vi "Solution Acquire Analyze Present.vi"() -> ()   [LabVIEW 2019]
panel:
  out "Difference":dbl
  out "Waveform Graph":dynamicdata(graph)
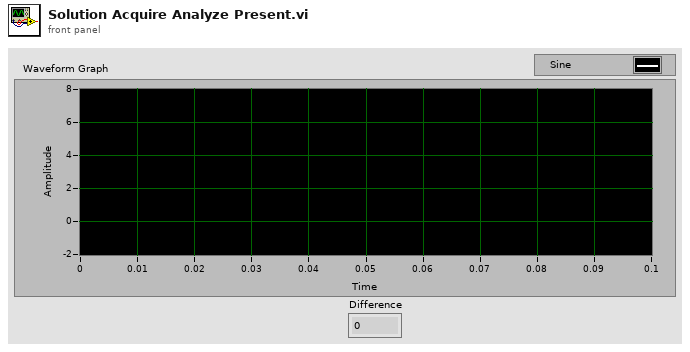
[diagram p1: front panel]
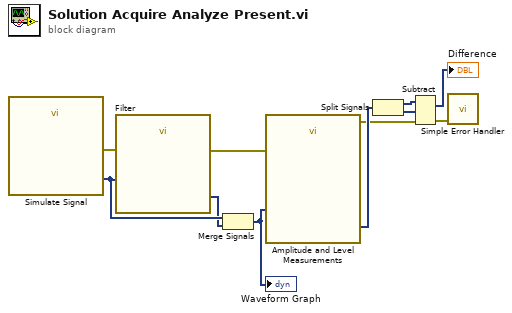
[diagram p0: block diagram]
diagram:
  n1 = call "Simulate Signal"() -> ("Sine"=w11:dynamicdata, "error out"=w4:errorcluster)  [unwired: 14 in]
  n2 = call "Filter"("error in (no error)"=w4, "Signal"=w11) -> ("error out"=w3:errorcluster, "Filtered Signal"=w10:dynamicdata)  [unwired: 8 in]
  n3 = Merge Signals(w11, w10) -> (w9:dynamicdata)
  "Waveform Graph" <- w9
  n4 = call "Amplitude and Level Measurements"("Signals"=w9, "error in (no error)"=w3) -> ("Peak to Peak"=w8:dynamicdata, "error out"=w2:errorcluster)  [unwired: 12 in]
  n5 = Split Signals(w8) -> (w7:dynamicdata, w6:dynamicdata)  [unwired: 2 in]
  n6 = Subtract(1:w6, 2:w7, 4:w2) -> (0:→"Difference":dynamicdata, 3:w1:errorcluster)
  n7 = call <vilib>:"Simple Error Handler.vi"("error in (no error)"=w1) -> ()  [unwired: 4 in, 5 out]
